vi "Create Callback User Events.vi"(8 "error in":errorcluster, 11 "MyEventGrid in":refnum<class "MyEventGrid.lvclass">) -> (0 "error out":errorcluster, 3 "MyEventGrid out":refnum<class "MyEventGrid.lvclass">)   [LabVIEW 2024, in "MyEventGrid.lvclass"]
uses:
  MyEventGrid.lvclass
  source/Cells/Cell Context/Cell Context.lvclass
  MyEventGrid.lvclass/MyEventGrid.ctl
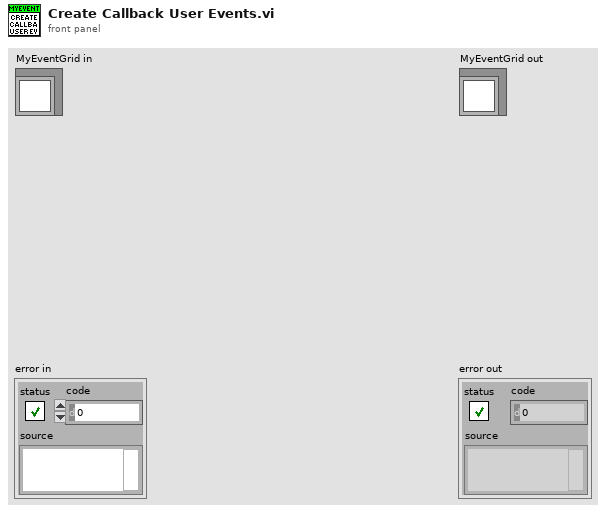
[diagram p1: front panel]
types:
  T1 = typedef "Rendezvous RefNum" = refnum<k1>
  T2 = cluster{"Context":refnum<class "Cell Context.lvclass">, "rendezvous":T1}
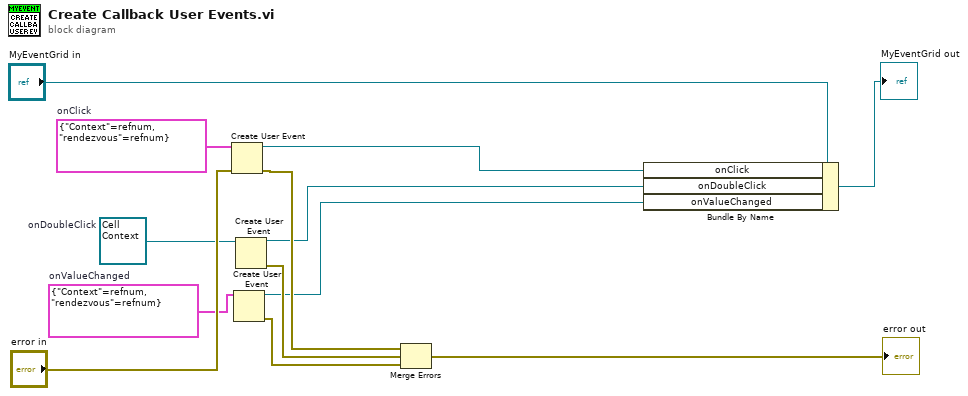
[diagram p0: block diagram]
diagram:
  w1 = T2 {"Context"=refnum, "rendezvous"=refnum}  # onValueChanged
  w2 = T2 {"Context"=refnum, "rendezvous"=refnum}  # onClick
  w8 = refnum<class "Cell Context.lvclass"> refnum  # onDoubleClick
  n1 = Create User Event(user event datatype=w2, error in="error in") -> (user event=w11:refnum<user-event>, error out=w7:errorcluster)
  n2 = Create User Event(user event datatype=w1) -> (user event=w4:refnum<user-event>, error out=w6:errorcluster)  [unwired: 1 in]
  n3 = Create User Event(user event datatype=w8) -> (user event=w5:refnum<user-event>, error out=w10:errorcluster)  [unwired: 1 in]
  n4 = Merge Errors(w7, w10, w6) -> (→"error out":errorcluster)
  n5 = Bundle By Name(cluster="MyEventGrid in", "onClick"=w11, "onDoubleClick"=w5, "onValueChanged"=w4) -> (→"MyEventGrid out":refnum<class "MyEventGrid.lvclass">)
